vi "Step_Forward.vi"(3 "error in":errorcluster, 4 "Data in":T1, 5 "Step control reference in":refnum<vi>) -> (0 "error out":errorcluster, 1 "Data out":T1, 2 "Step control reference out":refnum<vi>)   [LabVIEW 2017]
uses:
  Type_Defs/Data.ctl
  Type_Defs/Diagnostics.ctl
  Type_Defs/Systems.ctl
  Step_Vis/Steps.lvlib
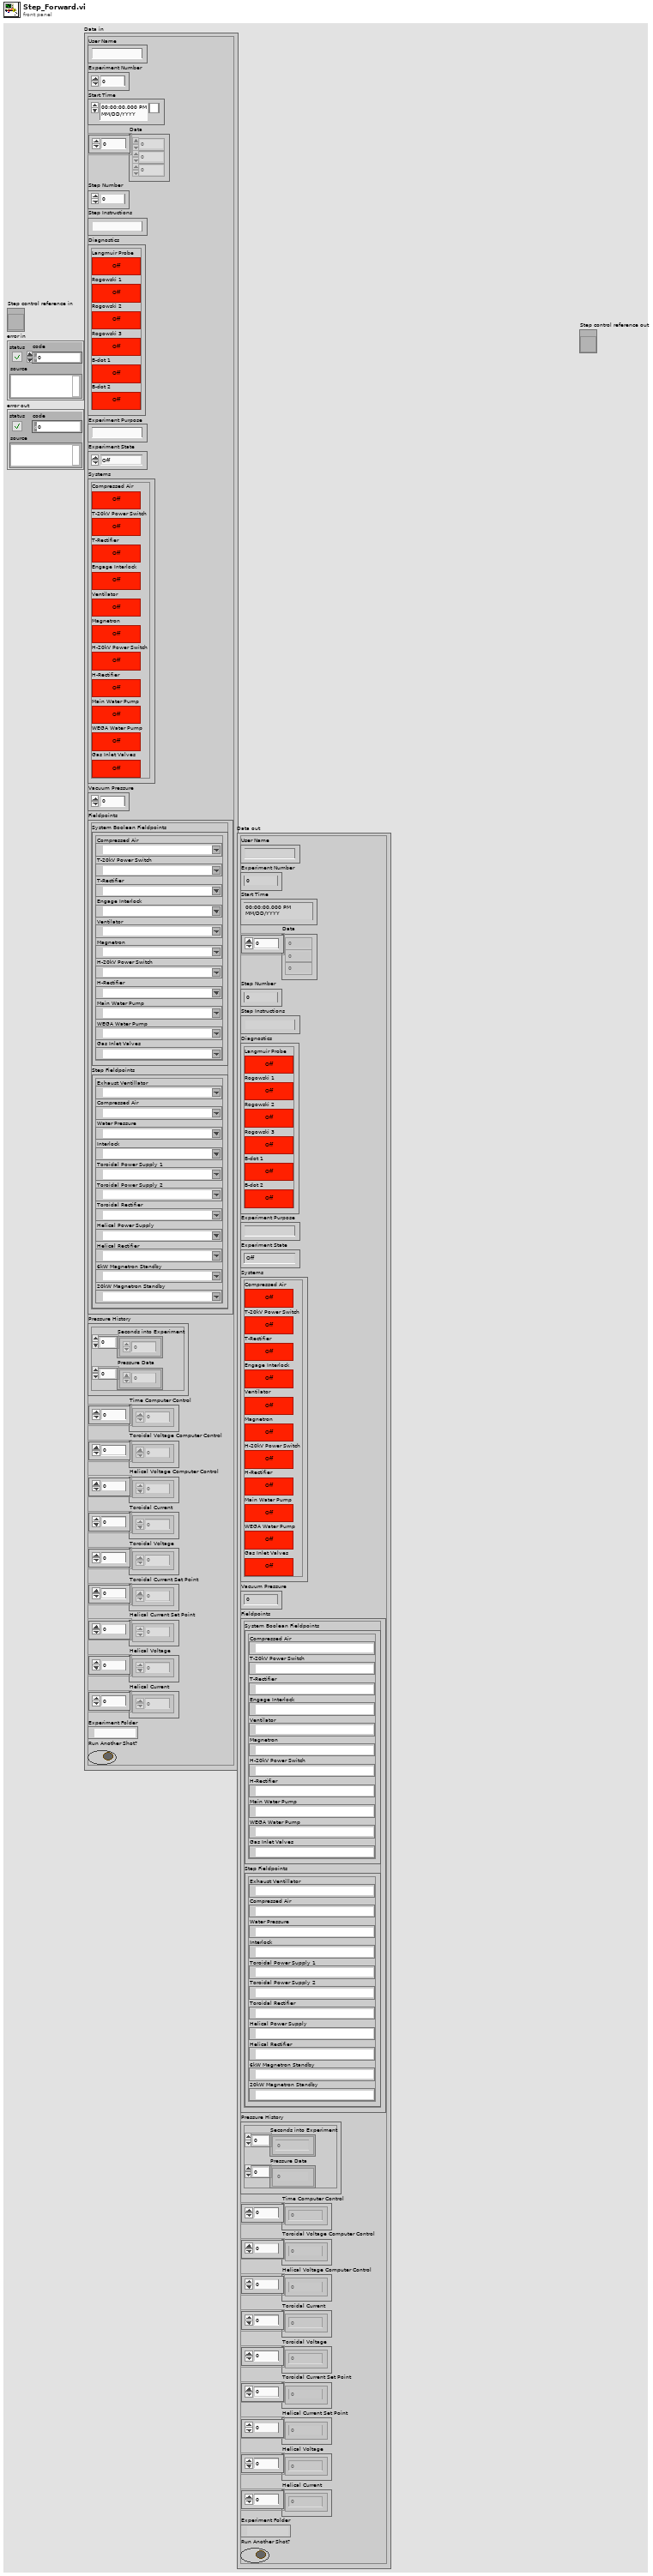
[diagram p1: front panel]
types:
  T1 = typedef "Data.ctl" = cluster{"User Name":string, "Experiment Number":i32, "Start Time":timestamp, "Data":dbl[], "Step Number":i32, "Step Instructions":string, "Diagnostics":T2, "Experiment Purpose":string, "Experiment State":enum16{"Off", "Setting Up", "Ready", "In Progress", "Shutting Down"}, "Systems":T3, "Vacuum Pressure":dbl, "Fieldpoints":cluster{"System Boolean Fieldpoints":cluster{"Compressed Air":refnum<k21>, "T-20kV Power Switch":refnum<k21>, "T-Rectifier":refnum<k21>, "Engage Interlock":refnum<k21>, "Ventilator":refnum<k21>, "Magnetron":refnum<k21>, "H-20kV Power Switch":refnum<k21>, "H-Rectifier":refnum<k21>, "Main Water Pump":refnum<k21>, "WEGA Water Pump":refnum<k21>, "Gas Inlet Valves":refnum<k21>}, "Step Fieldpoints":cluster{"Exhaust Ventillator":refnum<k21>, "Compressed Air":refnum<k21>, "Water Pressure":refnum<k21>, "Interlock":refnum<k21>, "Toroidal Power Supply 1":refnum<k21>, "Toroidal Power Supply 2":refnum<k21>, "Toroidal Rectifier":refnum<k21>, "Helical Power Supply":refnum<k21>, "Helical Rectifier":refnum<k21>, "6kW Magnetron Standby":refnum<k21>, "20kW Magnetron Standby":refnum<k21>}}, "Pressure History":cluster{"Seconds into Experiment":i32[], "Pressure Data":dbl[]}, "Time Computer Control":dbl[], "Toroidal Voltage Computer Control":dbl[], "Helical Voltage Computer Control":dbl[], "Toroidal Current":dbl[], "Toroidal Voltage":dbl[], "Toroidal Current Set Point":dbl[], "Helical Current Set Point":dbl[], "Helical Voltage":dbl[], "Helical Current":dbl[], "Experiment Folder":path, "Run Another Shot?":bool}
  T2 = typedef "Diagnostics.ctl" = cluster{"Langmuir Probe":bool, "Rogowski 1":bool, "Rogowski 2":bool, "Rogowski 3":bool, "B-dot 1":bool, "B-dot 2":bool}
  T3 = typedef "Systems.ctl" = cluster{"Compressed Air":bool, "T-20kV Power Switch":bool, "T-Rectifier":bool, "Engage Interlock":bool, "Ventilator":bool, "Magnetron":bool, "H-20kV Power Switch":bool, "H-Rectifier":bool, "Main Water Pump":bool, "WEGA Water Pump":bool, "Gas Inlet Valves":bool}
  T4 = enum16{"Off", "Setting Up", "Ready", "In Progress", "Shutting Down"}
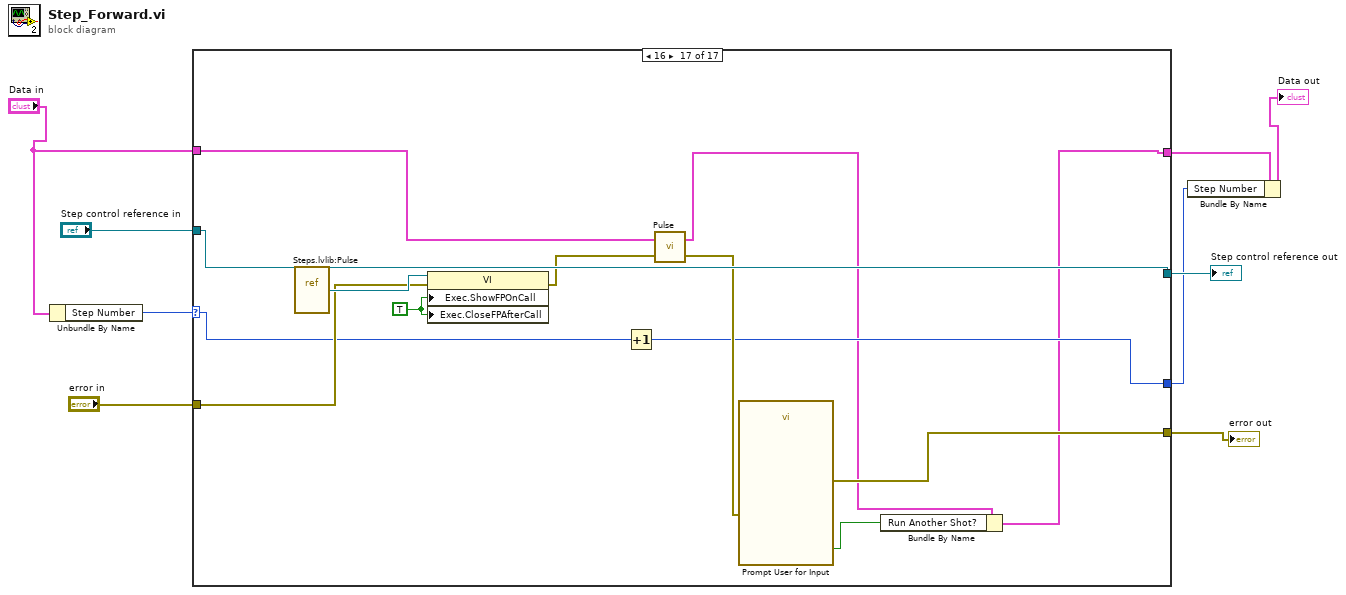
[diagram p0: block diagram]
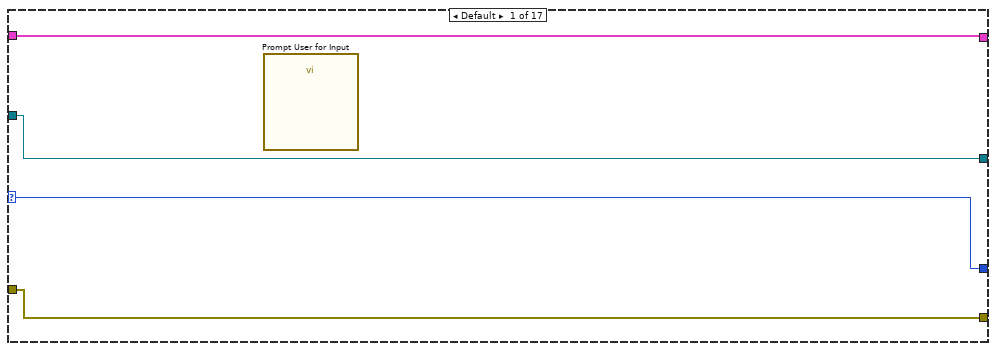
[diagram p2: hidden frame]
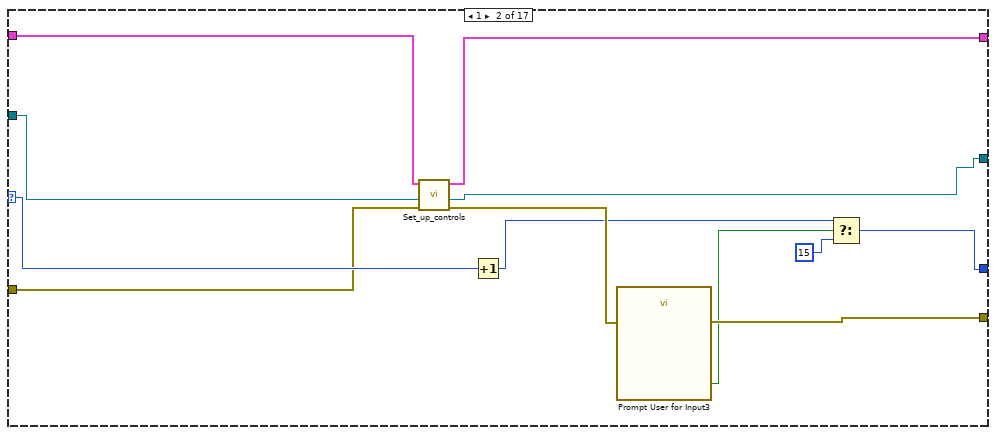
[diagram p3: hidden frame]
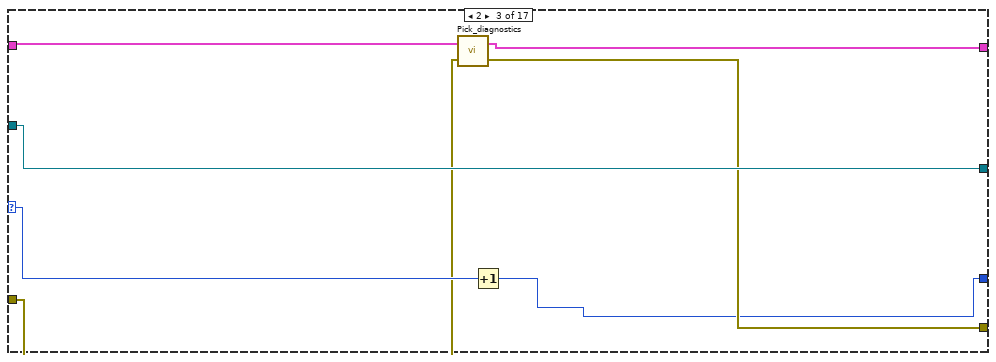
[diagram p4: hidden frame]
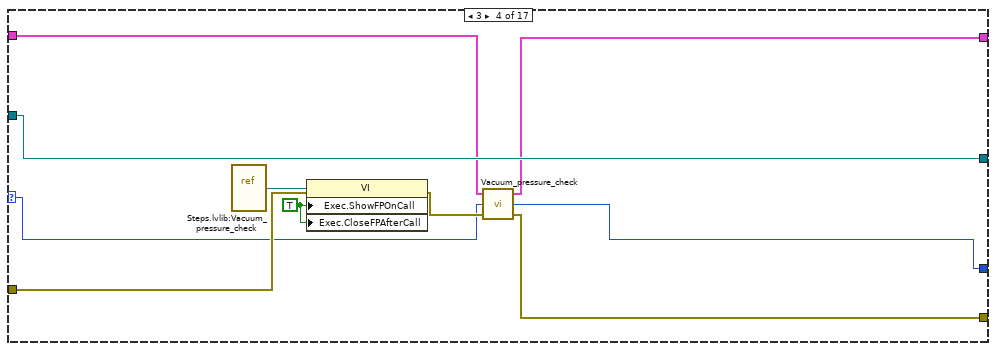
[diagram p5: hidden frame]
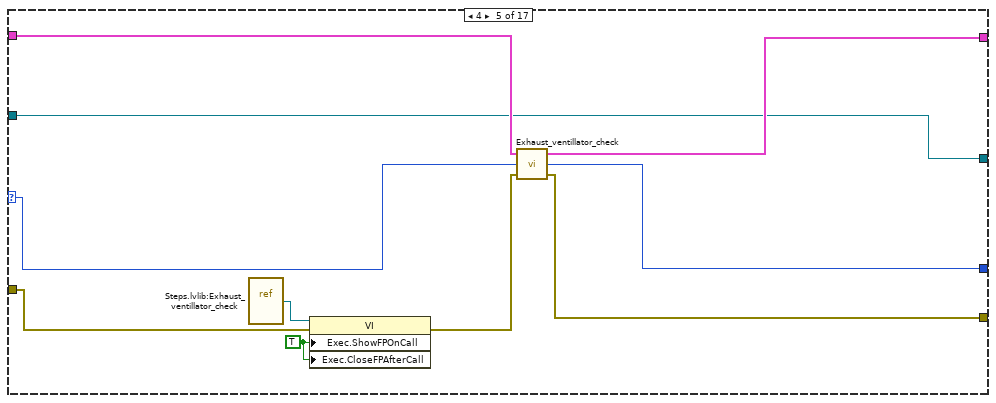
[diagram p6: hidden frame]
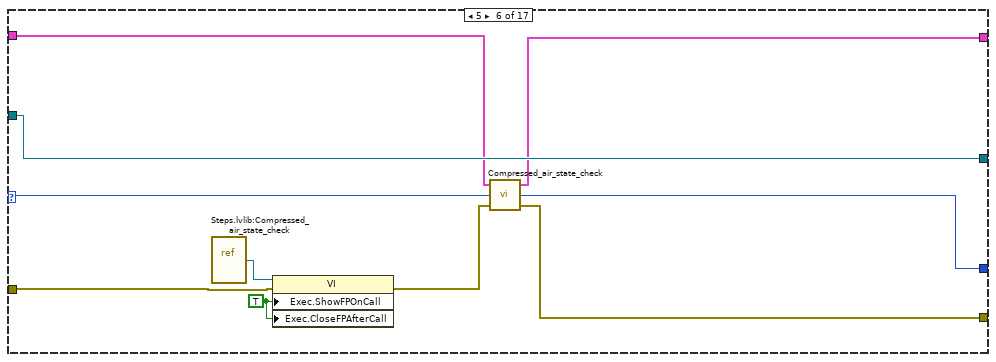
[diagram p7: hidden frame]
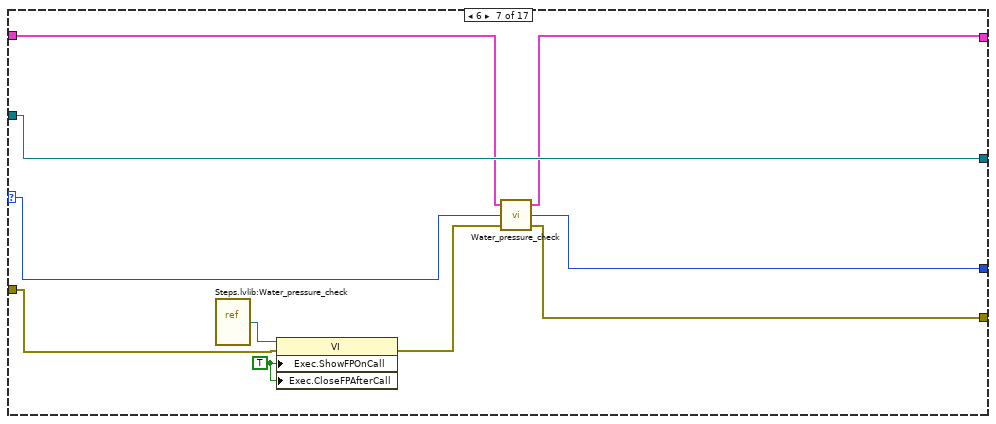
[diagram p8: hidden frame]
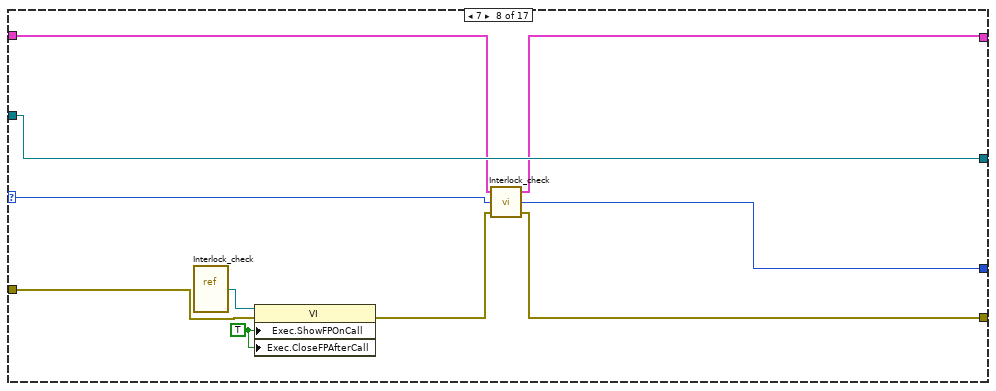
[diagram p9: hidden frame]
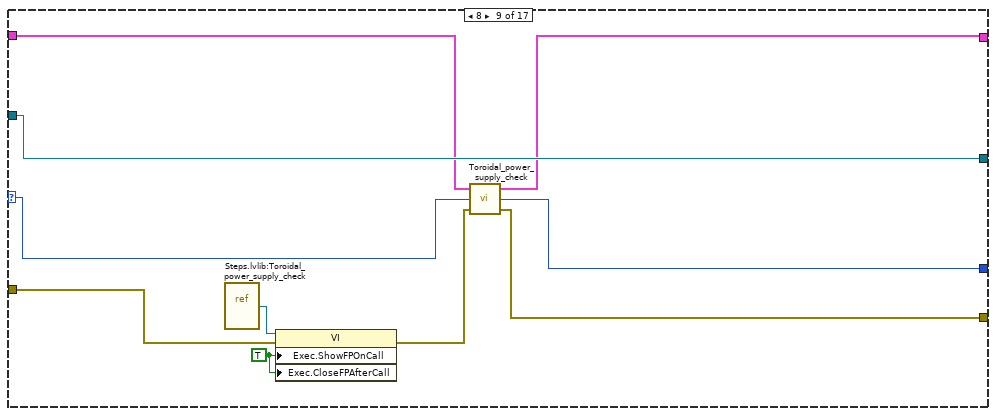
[diagram p10: hidden frame]
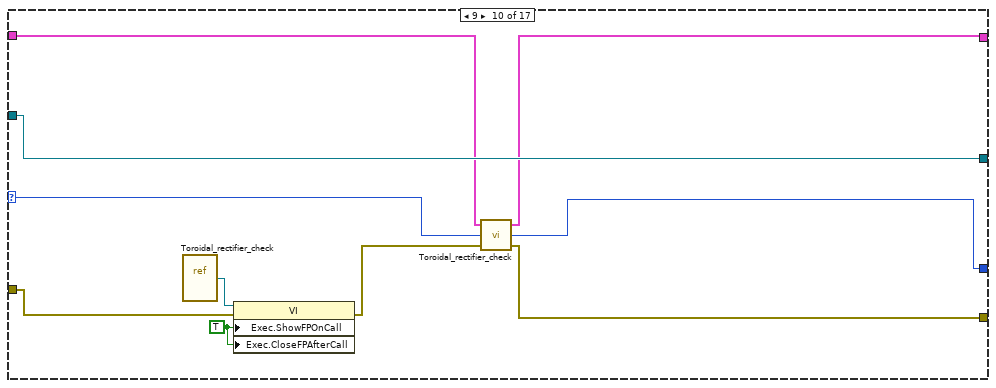
[diagram p11: hidden frame]
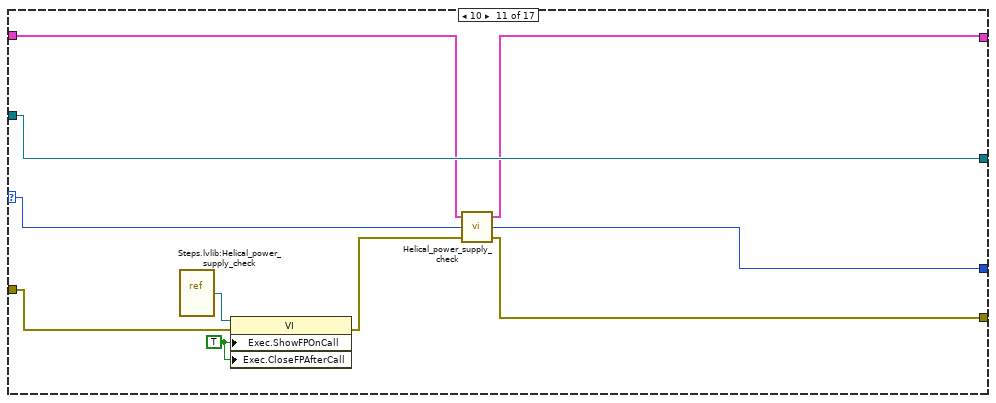
[diagram p12: hidden frame]
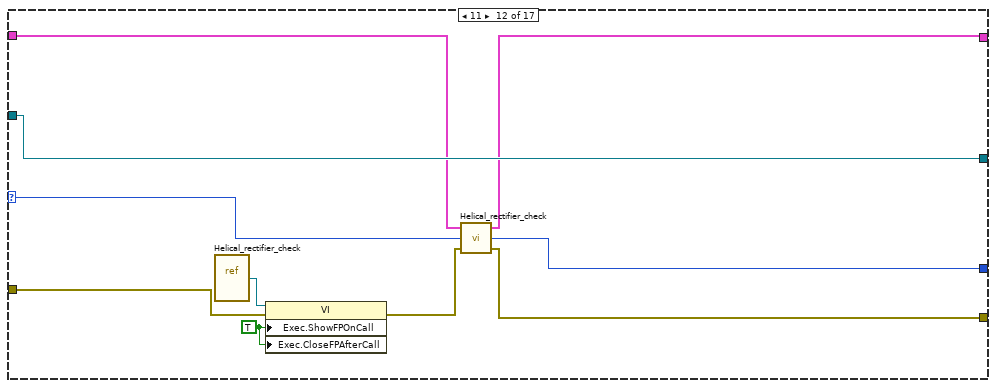
[diagram p13: hidden frame]
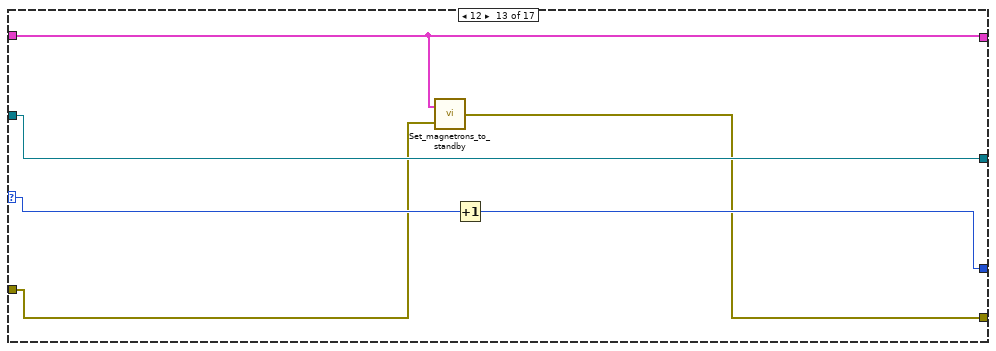
[diagram p14: hidden frame]
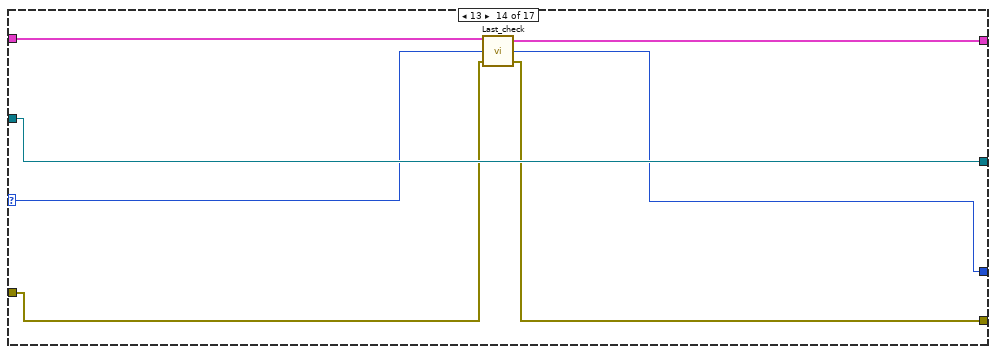
[diagram p15: hidden frame]
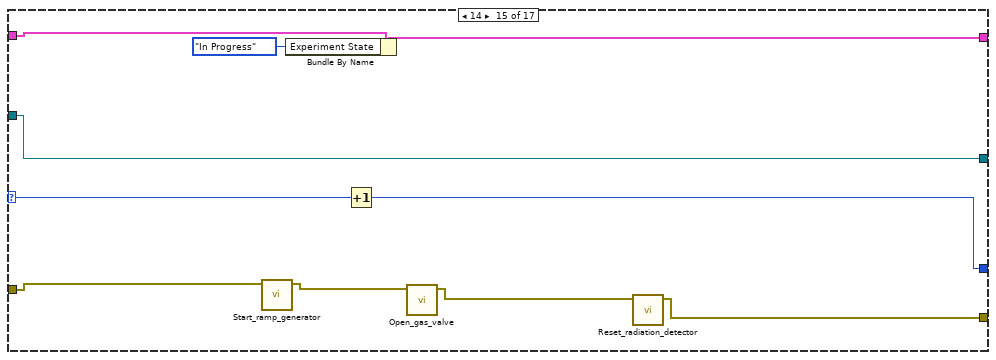
[diagram p16: hidden frame]
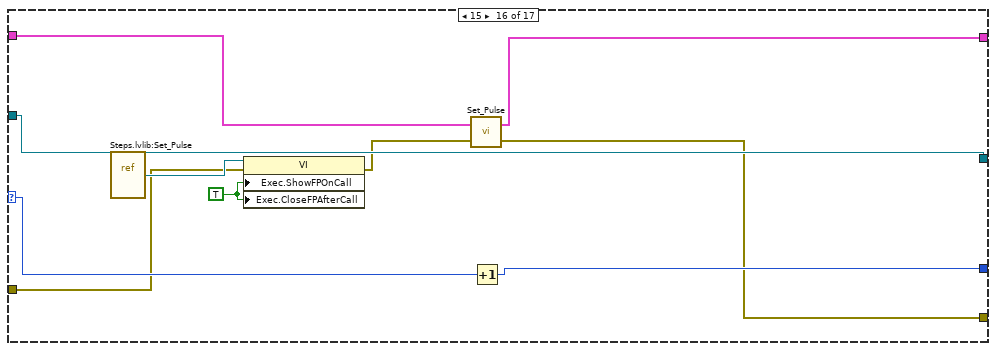
[diagram p17: hidden frame]
diagram:
  n1 = Unbundle By Name("Data in") -> ("Step Number"=w5:i32)
  n2 = case shown="16" w5 {
    selector: w5 -> [w12 w25 w32 w33 w49 w61 w69 w77 w89 w95 w106 w117 w126 w132 w143 w153 w159]
    tunnel: "Step control reference in" -> [w13 w23 w31 w42 w48 w62 w72 w82 w92 w102 w112 w122 w128 w135 w145 w155 w168]
    tunnel: [w13 w20 w31 w42 w48 w62 w72 w82 w92 w102 w112 w122 w128 w135 w145 w155 w168] -> w8
    tunnel: [w12 w15 w26 w34 w50 w57 w68 w78 w88 w96 w105 w116 w127 w131 w144 w154 w160] -> w3
    tunnel: "error in" -> [w11 w24 w27 w40 w45 w53 w63 w73 w86 w99 w109 w113 w124 w130 w142 w148 w164]
    tunnel: [w11 w18 w30 w38 w47 w58 w67 w79 w84 w97 w107 w115 w123 w129 w139 w146 w161] -> w6
    tunnel: "Data in" -> [w10 w22 w29 w36 w52 w59 w71 w81 w91 w94 w104 w119 w125 w134 w138 w150 w165]
    tunnel: [w10 w21 w28 w35 w51 w60 w70 w80 w90 w93 w103 w118 w125 w133 w137 w149 w157] -> w4
    frame Default {
      n3 = call "Prompt User for Input"() -> ()  [unwired: 18 in, 2 out]
    }
    frame 1 {
      n4 = call "Set_up_controls.vi"("error in"=w24, "reference"=w23, "Data in"=w22) -> ("error out"=w19:errorcluster, "reference out"=w20:refnum<vi>, "Data out"=w21:T1)  [unwired: 1 in, 1 out]
      n5 = Increment(x=w25) -> (x+1=w16:i32)
      n6 = call "Prompt User for Input3"("error in (no error)"=w19) -> ("Setup"=w14:bool, "error out"=w18:errorcluster)  [unwired: 16 in, 1 out]
      n7 = Select(t=w16, s=w14, f=15) -> (s? t:f=w15:i32)
    }
    frame 2 {
      n8 = call "Pick_diagnostics.vi"("error in (no error)"=w27, "Data In"=w29) -> ("error out"=w30:errorcluster, "Data Out"=w28:T1)
      n9 = Increment(x=w32) -> (x+1=w26:i32)
    }
    frame 3 {
      w37 = TRUE ("Execution:Show Front Panel On Call")
      n10 = vi-ref "Steps.lvlib:Vacuum_pressure_check.vi"() -> (w41:refnum<vi>)
      n11 = property class="VI"(reference=w41, error in=w40, "Exec.ShowFPOnCall"=w37, "Exec.CloseFPAfterCall"=w37) -> (error out=w39:errorcluster)  [unwired: 1 out]
      n12 = call "Vacuum_pressure_check.vi"("error in"=w39, "Step Number in"=w33, "Data in"=w36) -> ("error out"=w38:errorcluster, "Step Number out"=w34:i32, "Data out"=w35:T1)
    }
    frame 4 {
      w46 = TRUE ("Execution:Show Front Panel On Call")
      n13 = vi-ref "Steps.lvlib:Exhaust_ventillator_check.vi"() -> (w43:refnum<vi>)
      n14 = property class="VI"(reference=w43, error in=w45, "Exec.ShowFPOnCall"=w46, "Exec.CloseFPAfterCall"=w46) -> (error out=w44:errorcluster)  [unwired: 1 out]
      n15 = call "Exhaust_ventillator_check.vi"("error in"=w44, "Step Number in"=w49, "Data in"=w52) -> ("error out"=w47:errorcluster, "Step Number out"=w50:i32, "Data out"=w51:T1)
    }
    frame 5 {
      w56 = TRUE ("Execution:Show Front Panel On Call")
      n16 = vi-ref "Steps.lvlib:Compressed_air_state_check.vi"() -> (w55:refnum<vi>)
      n17 = property class="VI"(reference=w55, error in=w53, "Exec.ShowFPOnCall"=w56, "Exec.CloseFPAfterCall"=w56) -> (error out=w54:errorcluster)  [unwired: 1 out]
      n18 = call "Compressed_air_state_check.vi"("error in"=w54, "Step Number in"=w61, "Data in"=w59) -> ("error out"=w58:errorcluster, "Step Number out"=w57:i32, "Data out"=w60:T1)
    }
    frame 6 {
      w66 = TRUE ("Execution:Show Front Panel On Call")
      n19 = vi-ref "Steps.lvlib:Water_pressure_check.vi"() -> (w65:refnum<vi>)
      n20 = property class="VI"(reference=w65, error in=w63, "Exec.ShowFPOnCall"=w66, "Exec.CloseFPAfterCall"=w66) -> (error out=w64:errorcluster)  [unwired: 1 out]
      n21 = call "Water_pressure_check.vi"("error in"=w64, "Step Number in"=w69, "Data in"=w71) -> ("error out"=w67:errorcluster, "Step Number out"=w68:i32, "Data out"=w70:T1)
    }
    frame 7 {
      w75 = TRUE ("Execution:Show Front Panel On Call")
      n22 = vi-ref "Interlock_check.vi"() -> (w76:refnum<vi>)
      n23 = property class="VI"(reference=w76, error in=w73, "Exec.ShowFPOnCall"=w75, "Exec.CloseFPAfterCall"=w75) -> (error out=w74:errorcluster)  [unwired: 1 out]
      n24 = call "Interlock_check.vi"("error in"=w74, "Step Number in"=w77, "Data in"=w81) -> ("error out"=w79:errorcluster, "Step Number out"=w78:i32, "Data out"=w80:T1)
    }
    frame 8 {
      w87 = TRUE ("Execution:Show Front Panel On Call")
      n25 = vi-ref "Steps.lvlib:Toroidal_power_supply_check.vi"() -> (w83:refnum<vi>)
      n26 = property class="VI"(reference=w83, error in=w86, "Exec.ShowFPOnCall"=w87, "Exec.CloseFPAfterCall"=w87) -> (error out=w85:errorcluster)  [unwired: 1 out]
      n27 = call "Toroidal_power_supply_check.vi"("error in"=w85, "Step Number in"=w89, "Data in"=w91) -> ("error out"=w84:errorcluster, "Step Number out"=w88:i32, "Data out"=w90:T1)
    }
    frame 9 {
      w101 = TRUE ("Execution:Show Front Panel On Call")
      n28 = vi-ref "Toroidal_rectifier_check.vi"() -> (w100:refnum<vi>)
      n29 = property class="VI"(reference=w100, error in=w99, "Exec.ShowFPOnCall"=w101, "Exec.CloseFPAfterCall"=w101) -> (error out=w98:errorcluster)  [unwired: 1 out]
      n30 = call "Toroidal_rectifier_check.vi"("error in"=w98, "Step Number in"=w95, "Data in"=w94) -> ("error out"=w97:errorcluster, "Step Number out"=w96:i32, "Data out"=w93:T1)
    }
    frame 10 {
      w110 = TRUE ("Execution:Show Front Panel On Call")
      n31 = vi-ref "Steps.lvlib:Helical_power_supply_check.vi"() -> (w111:refnum<vi>)
      n32 = property class="VI"(reference=w111, error in=w109, "Exec.ShowFPOnCall"=w110, "Exec.CloseFPAfterCall"=w110) -> (error out=w108:errorcluster)  [unwired: 1 out]
      n33 = call "Helical_power_supply_check.vi"("error in"=w108, "Step Number in"=w106, "Data in"=w104) -> ("error out"=w107:errorcluster, "Step Number out"=w105:i32, "Data out"=w103:T1)
    }
    frame 11 {
      w120 = TRUE ("Execution:Show Front Panel On Call")
      n34 = vi-ref "Helical_rectifier_check.vi"() -> (w121:refnum<vi>)
      n35 = property class="VI"(reference=w121, error in=w113, "Exec.ShowFPOnCall"=w120, "Exec.CloseFPAfterCall"=w120) -> (error out=w114:errorcluster)  [unwired: 1 out]
      n36 = call "Helical_rectifier_check.vi"("error in"=w114, "Step Number in"=w117, "Data in"=w119) -> ("error out"=w115:errorcluster, "Step Number out"=w116:i32, "Data out"=w118:T1)
    }
    frame 12 {
      n37 = call "Set_magnetrons_to_standby.vi"("error in"=w124, "Data in"=w125) -> ("error out"=w123:errorcluster)
      n38 = Increment(x=w126) -> (x+1=w127:i32)
    }
    frame 13 {
      n39 = call "Last_check.vi"("error in"=w130, "Step Number in"=w132, "Data in"=w134) -> ("error out"=w129:errorcluster, "Step Number out"=w131:i32, "Data out"=w133:T1)
    }
    frame 14 {
      n40 = call "Start_ramp_generator.vi"("error in"=w142) -> ("error out"=w141:errorcluster)  [unwired: 10 in]
      n41 = Bundle By Name(cluster=w138, "Experiment State"=T4."In Progress") -> (w137:T1)
      n42 = Increment(x=w143) -> (x+1=w144:i32)
      n43 = call "Open_gas_valve.vi"("error in"=w141) -> ("error out"=w140:errorcluster)  [unwired: 10 in]
      n44 = call "Reset_radiation_detector.vi"("error in"=w140) -> ("error out"=w139:errorcluster)  [unwired: 10 in]
    }
    frame 15 {
      w152 = TRUE ("Execution:Show Front Panel On Call")
      n45 = vi-ref "Steps.lvlib:Set_Pulse.vi"() -> (w151:refnum<vi>)
      n46 = property class="VI"(reference=w151, error in=w148, "Exec.ShowFPOnCall"=w152, "Exec.CloseFPAfterCall"=w152) -> (error out=w147:errorcluster)  [unwired: 1 out]
      n47 = call "Set_Pulse.vi"("error in"=w147, "Data in"=w150) -> ("error out"=w146:errorcluster, "Data out"=w149:T1)
      n48 = Increment(x=w153) -> (x+1=w154:i32)
    }
    frame 16 {
      w167 = TRUE ("Execution:Show Front Panel On Call")
      n49 = vi-ref "Steps.lvlib:Pulse.vi"() -> (w166:refnum<vi>)
      n50 = property class="VI"(reference=w166, error in=w164, "Exec.ShowFPOnCall"=w167, "Exec.CloseFPAfterCall"=w167) -> (error out=w163:errorcluster)  [unwired: 1 out]
      n51 = Increment(x=w159) -> (x+1=w160:i32)
      n52 = call "Pulse.vi"("error in"=w163, "Data in"=w165) -> ("error out"=w162:errorcluster, "Data out"=w158:T1)
      n53 = call "Prompt User for Input"("error in (no error)"=w162) -> ("Run New Shot"=w156:bool, "error out"=w161:errorcluster)  [unwired: 16 in, 1 out]
      n54 = Bundle By Name(cluster=w158, "Run Another Shot?"=w156) -> (w157:T1)
    }
  }
  "Step control reference out" <- w8
  "error out" <- w6
  n55 = Bundle By Name(cluster=w4, "Step Number"=w3) -> (→"Data out":T1)
